vi "area.vi"(8 "error in (no error)":errorcluster, 11 "Input":string="34,45,89") -> (0 "error out":errorcluster, 3 "Output":string)   [LabVIEW 2014]
uses:
  <userlib>/Nanonis Prog Interface V5/Nanonis Prog Interface.lvlib
panel:
  out "size(s)":i32=3
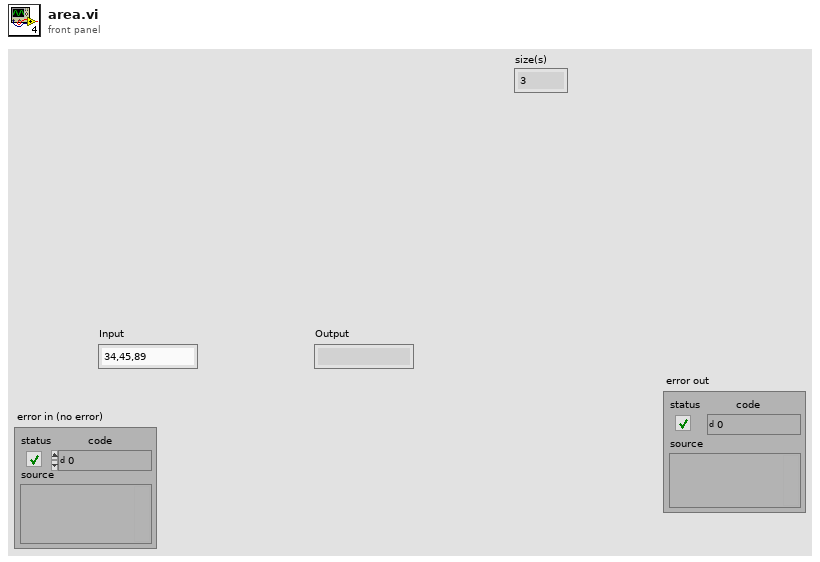
[diagram p1: front panel]
types:
  T1 = enum8{"Group 1", "Group 2", "Group 3", "Group 4", "Group 5", "Group 6"}
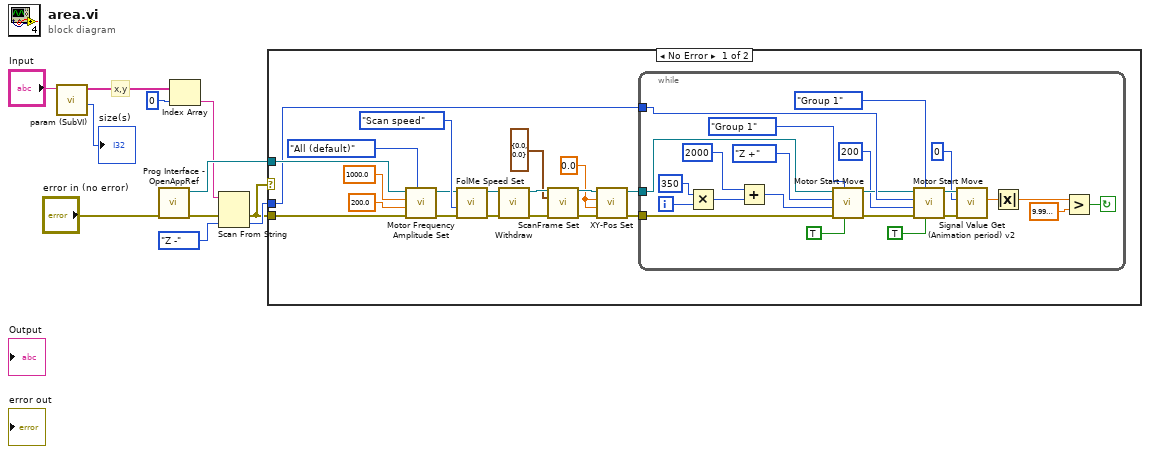
[diagram p0: block diagram]
diagram:
  # "x,y"
  n1 = call <userlib>:"param (SubVI).vi"("Input"="Input") -> ("num"=→"size(s)":i32, "Array"=w7:string[])  [unwired: 8 in, 1 out]
  n2 = call <userlib>:"Prog Interface - OpenAppRef.vi"("Error in (no error)"="error in (no error)") -> ("Error out"=w2:errorcluster, "Application reference"=w8:refnum<vi>)  [unwired: 5 in]
  n3 = Index Array(array=w7, index=0) -> (element=w5:string)
  n4 = Scan From String(input string=w5, error in=w2, default 1=enum16{"X +", "X -", "Y +", "Y -", "Z +", "Z -"}."Z -" ("Direction")) -> (error out=w1:errorcluster, output 1=w3:enum16{"X +", "X -", "Y +", "Y -", "Z +", "Z -"})  [unwired: 2 in, 2 out]
  n5 = case shown="No Error" w1 {
    tunnel: w8 -> [w18 _]
    tunnel: w3 -> [w16 _]
    tunnel: w1 -> [w13 _]
    frame No Error {
      w25 = sgl 0.0 ("X (m)")
      n6 = call <userlib>:"Motor Frequency Amplitude Set.vi"("Axis (All)"=enum16{"All (default)", "X", "Y", "Z"}."All (default)", "Error in (no error)"=w13, "Amplitude (V) (NaN=no change)"=sgl 200.0, "Frequency (Hz) (NaN=no change)"=sgl 1000.0, "Application ref in"=w18) -> ("Error out"=w12:errorcluster, "Application ref out"=w17:refnum<vi>)  [unwired: 5 in]
      n7 = call <userlib>:"FolMe Speed Set.vi"("error in (no error)"=w12, "Speed Setting (Custom)"=enum32{"Scan speed", "Custom speed"}."Scan speed", "Application ref in"=w17) -> ("error out"=w22:errorcluster, "Application ref out"=w23:refnum<vi>)  [unwired: 5 in]
      n8 = call <userlib>:"Withdraw.vi"("Error in (no error)"=w22, "Application ref in"=w23) -> ("Error out"=w29:errorcluster, "Application ref out"=w30:refnum<vi>)  [unwired: 8 in]
      n9 = call <userlib>:"ScanFrame Set.vi"("Application ref in"=w30, "Center coordinates (m)"=cluster{"Xc":sgl, "Yc":sgl} {"Xc"=0.0, "Yc"=0.0}, "error in (no error)"=w29) -> ("Application ref out"=w26:refnum<vi>, "error out"=w27:errorcluster)  [unwired: 11 in]
      n10 = call <userlib>:"XY-Pos Set.vi"("error in (no error)"=w27, "Y (m)"=w25, "X (m)"=w25, "Application ref in"=w26) -> ("error out"=w14:errorcluster, "Application ref out"=w15:refnum<vi>)  [unwired: 4 in]
      n11 = while {
        tunnel: w16 -> [w53]
        tunnel: w15 -> [w52]
        tunnel: w14 -> [w51]
        i -> [w34]
        stop <- w36 continue-if-true
        n12 = Multiply(x=350, y=w34) -> (x*y=w32:i32)
        n13 = Add(x=u16 2000 ("Number of steps"), y=w32) -> (x+y=w35:i32)
        n14 = call <userlib>:"Motor Start Move.vi"("Wait until finished? (F)"=TRUE, "Group"=T1."Group 1", "Error in (no error)"=w51, "Number of steps"=w35, "Direction"=enum16{"X +", "X -", "Y +", "Y -", "Z +", "Z -"}."Z +", "Application ref in"=w52) -> ("Error out"=w46:errorcluster, "Application ref out"=w47:refnum<vi>)  [unwired: 3 in]
        n15 = call <userlib>:"Motor Start Move.vi"("Wait until finished? (F)"=TRUE, "Group"=T1."Group 1", "Error in (no error)"=w46, "Number of steps"=u16 200, "Direction"=w53, "Application ref in"=w47) -> ("Error out"=w40:errorcluster, "Application ref out"=w42:refnum<vi>)  [unwired: 3 in]
        n16 = call <userlib>:"Signal Value Get (Animation period) v2.vi"("error in (no error)"=w40, "Signal index (0-79)"=i8 0, "Application ref in"=w42) -> ("Signal value"=w39:sgl)  [unwired: 5 in, 2 out]
        n17 = Absolute Value(x=w39) -> (abs(x)=w37:sgl)
        n18 = Greater?(x=w37, y=sgl 1e-09) -> (0:w36:bool)
      }
    }
    frame Error {
    }
  }
